vi "CSM - Load Configuration Variables From String.vi"(5 "Section Postfix (\"\")":string, 8 "error in (no error)":errorcluster, 9 "Configuration String":string="[section]\nkey = Value") -> (2 "error out":errorcluster)   [LabVIEW 2017, in "INI-Static-Variable-Support.lvlib"]
doc: "Loads configuration variables from a specified string. If the section name postfix is not empty, the loaded section names will have this postfix appended.\n\n<b>Section Postfix (\"\")</b> is primarily used when loading multiple configuration files that have identical sections. For example, two configuration files `Hardware1.ini` and `Hardware2.ini` both have a section named `Serial` with identical internal keys indicating serial port configuration. In this case, the configuration in the file loaded later would overwrite the configuration in the file loaded earlier. Using <b>Section Postfix (\"\")</b> prevents section name conflicts.\n\n<b>Reference Example</b>: `8. import Configuration From String.vi`.\n\n\n> [!NOTE] <b>CSM INI-Variable Configuration File Path</b>\n>\n> - <b>Development State</b>: The first INI configuration file found in the Application Directory. If no configuration file exists, it defaults to `csm-app.ini`.\n> - <b>Post-Compilation</b>: An INI configuration file in the same directory as the executable file, with the same name as the executable. LabVIEW automatically generates this file after compilation.\n> - Supports loading multiple configuration files. Configuration items in files loaded later will overwrite identical items in previously loaded files.\n> - Configuration files can use the `[__include]` section to reference other configuration files.\n> - Supports both relative and absolute paths.\n> - Relative paths are relative to the path of the current configuration file.\n> - The name of the configuration file in the `[__include]` section is not critical, as long as the path is correct.\n> - To avoid circular references, the same configuration file will be automatically ignored if loaded a second time.\n\n\n-- <b>Controls</b> --\n- <b>Configuration String</b>: Configuration string.\n- <b>Section Postfix (\"\")</b>: Section name postfix."
uses:
  INI-Static-Variable-Support.lvlib
  _Support/_fgv-oper.ctl
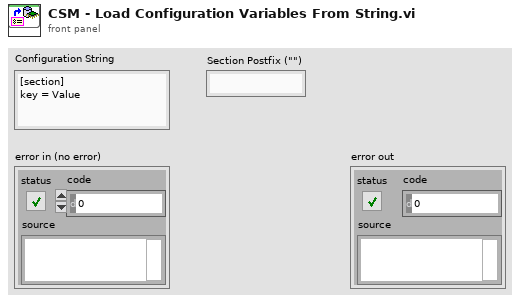
[diagram p1: front panel]
types:
  T1 = typedef "INI-Static-Variable-Support.lvlib/_fgv-oper.ctl" = enum16{"Read", "Write", "Sync", "Sessions", "List Keys", "Load", "List Files", "List Variables", "List Permanent Variables", "Mark Temp Variable as Permenent", "unload", "INIConfig(Memory)", "Reset", "Restore Variable Value", "Load From String"}
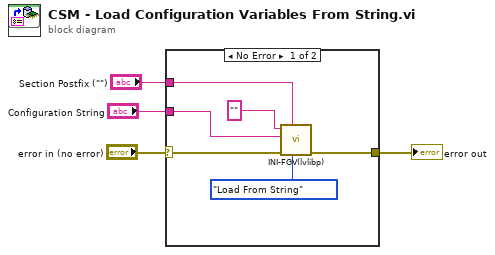
[diagram p0: block diagram]
diagram:
  n1 = case shown="No Error" "error in (no error)" {
    selector: "error in (no error)" -> [w9 w11]
    tunnel: "Configuration String" -> [w6 _]
    tunnel: [w8 w11] -> w2
    tunnel: "Section Postfix (\"\")" -> [w7 _]
    frame No Error {
      n2 = call "INI-FGV(lvlibp).vi"("Enum"=_fgv-oper."Load From String", "Prefered Section"=w7, "error IN"=w9, ">> Default Value >>"=w6, ">> Variable Name >>"="") -> ("error out"=w8:errorcluster)  [unwired: 3 in, 3 out]
    }
    frame Error {
    }
  }
  "error out" <- w2
